vi "Diff_Drive_System_Dash_Write.vi"   [LabVIEW 2019]
uses:
  Diff_Drive_System_Globals.vi
  <vilib>/Rock Robotics/Network Tables/NT Write Numeric Array.vi
  <vilib>/Rock Robotics/Network Tables/NT Write Number.vi
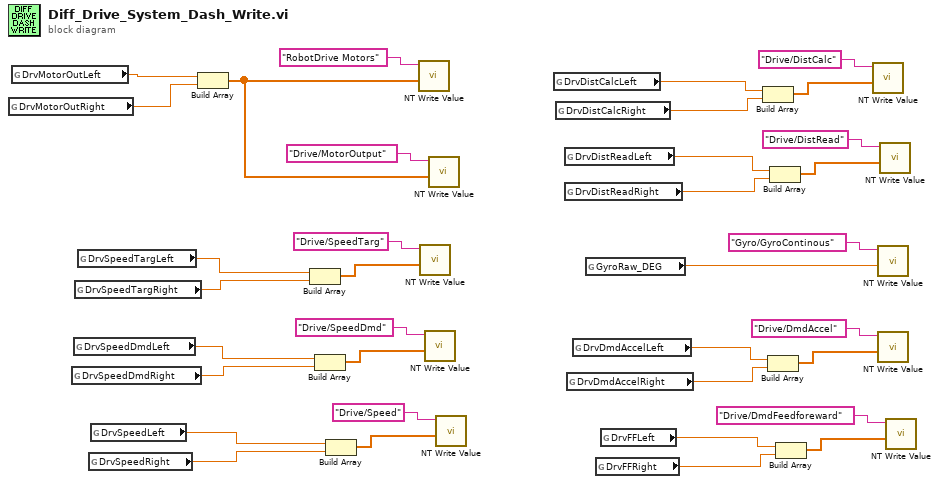
[diagram p0: block diagram]
diagram:
  n1 = global read "Diff_Drive_System_Globals.vi" "DrvMotorOutRight"() -> (w17:dbl)
  n2 = global read "Diff_Drive_System_Globals.vi" "DrvMotorOutLeft"() -> (w18:dbl)
  n3 = global read "Diff_Drive_System_Globals.vi" "DrvSpeedDmdRight"() -> (w12:dbl)
  n4 = global read "Diff_Drive_System_Globals.vi" "DrvSpeedDmdLeft"() -> (w13:dbl)
  n5 = global read "Diff_Drive_System_Globals.vi" "DrvSpeedTargRight"() -> (w14:dbl)
  n6 = global read "Diff_Drive_System_Globals.vi" "DrvSpeedTargLeft"() -> (w15:dbl)
  n7 = global read "Diff_Drive_System_Globals.vi" "DrvSpeedRight"() -> (w10:dbl)
  n8 = global read "Diff_Drive_System_Globals.vi" "DrvSpeedLeft"() -> (w11:dbl)
  n9 = Build Array(w18, w17) -> (w16:dbl[])
  n10 = Build Array(w15, w14) -> (w21:dbl[])
  n11 = Build Array(w13, w12) -> (w23:dbl[])
  n12 = Build Array(w11, w10) -> (w25:dbl[])
  n13 = call-poly <vilib>:"NT Write Value.vi"("Numeric Array"=w16, "Name"="RobotDrive Motors") -> ()  [unwired: 9 in, 1 out]
  n14 = call-poly <vilib>:"NT Write Value.vi"("Numeric Array"=w21, "Name"="Drive/SpeedTarg") -> ()  [unwired: 9 in, 1 out]
  n15 = call-poly <vilib>:"NT Write Value.vi"("Numeric Array"=w23, "Name"="Drive/SpeedDmd") -> ()  [unwired: 9 in, 1 out]
  n16 = call-poly <vilib>:"NT Write Value.vi"("Numeric Array"=w16, "Name"="Drive/MotorOutput") -> ()  [unwired: 9 in, 1 out]
  n17 = call-poly <vilib>:"NT Write Value.vi"("Numeric Array"=w25, "Name"="Drive/Speed") -> ()  [unwired: 9 in, 1 out]
  n18 = global read "Diff_Drive_System_Globals.vi" "DrvDistCalcLeft"() -> (w9:dbl)
  n19 = global read "Diff_Drive_System_Globals.vi" "DrvDistCalcRight"() -> (w8:dbl)
  n20 = global read "Diff_Drive_System_Globals.vi" "DrvDistReadLeft"() -> (w7:dbl)
  n21 = global read "Diff_Drive_System_Globals.vi" "DrvDistReadRight"() -> (w6:dbl)
  n22 = global read "Diff_Drive_System_Globals.vi" "DrvDmdAccelRight"() -> (w3:dbl)
  n23 = global read "Diff_Drive_System_Globals.vi" "DrvDmdAccelLeft"() -> (w4:dbl)
  n24 = global read "Diff_Drive_System_Globals.vi" "GyroRaw_DEG"() -> (w5:dbl)
  n25 = global read "Diff_Drive_System_Globals.vi" "DrvFFRight"() -> (w1:dbl)
  n26 = global read "Diff_Drive_System_Globals.vi" "DrvFFLeft"() -> (w2:dbl)
  n27 = Build Array(w9, w8) -> (w27:dbl[])
  n28 = Build Array(w4, w3) -> (w32:dbl[])
  n29 = Build Array(w7, w6) -> (w29:dbl[])
  n30 = Build Array(w2, w1) -> (w34:dbl[])
  n31 = call-poly <vilib>:"NT Write Value.vi"("Numeric Array"=w27, "Name"="Drive/DistCalc") -> ()  [unwired: 9 in, 1 out]
  n32 = call-poly <vilib>:"NT Write Value.vi"("Numeric"=w5, "Name"="Gyro/GyroContinous") -> ()  [unwired: 9 in, 1 out]
  n33 = call-poly <vilib>:"NT Write Value.vi"("Numeric Array"=w32, "Name"="Drive/DmdAccel") -> ()  [unwired: 9 in, 1 out]
  n34 = call-poly <vilib>:"NT Write Value.vi"("Numeric Array"=w29, "Name"="Drive/DistRead") -> ()  [unwired: 9 in, 1 out]
  n35 = call-poly <vilib>:"NT Write Value.vi"("Numeric Array"=w34, "Name"="Drive/DmdFeedforeward") -> ()  [unwired: 9 in, 1 out]
